vi "Brute Force Measurment SubVI.vi"(0 "Data Pin Task In":refnum<k21>, 1 "Sync Pin Task In":refnum<k21>, 2 "Write Pin Task In":refnum<k21>, 3 "Clear Pin Task In":refnum<k21>, 4 "Barcodes in":string[](array[string]), 5 "Channel # in":i32, 6 "Number of Active tubes":i32, 7 "error in (no error)":errorcluster, 9 "BoardHandle in":T1) -> (11 "Actual Voltage Level (V) 2":dbl format="%#_13g", 12 "Individual Tube Current (Nano Amps)":dbl[](array[numeric]), 13 "Failed Tubes":string[](array[string]), 14 "Data Pin Task Out":refnum<k21>, 15 "Sync Pin Task Out":refnum<k21>, 16 "Write Pin Task Out":refnum<k21>, 17 "Clear Pin Task Out":refnum<k21>, 18 "error out":errorcluster, 19 "BoardHandle out":T1)   [LabVIEW 2020]
panel:
  # "Pin in."
  # "Output pin positions"
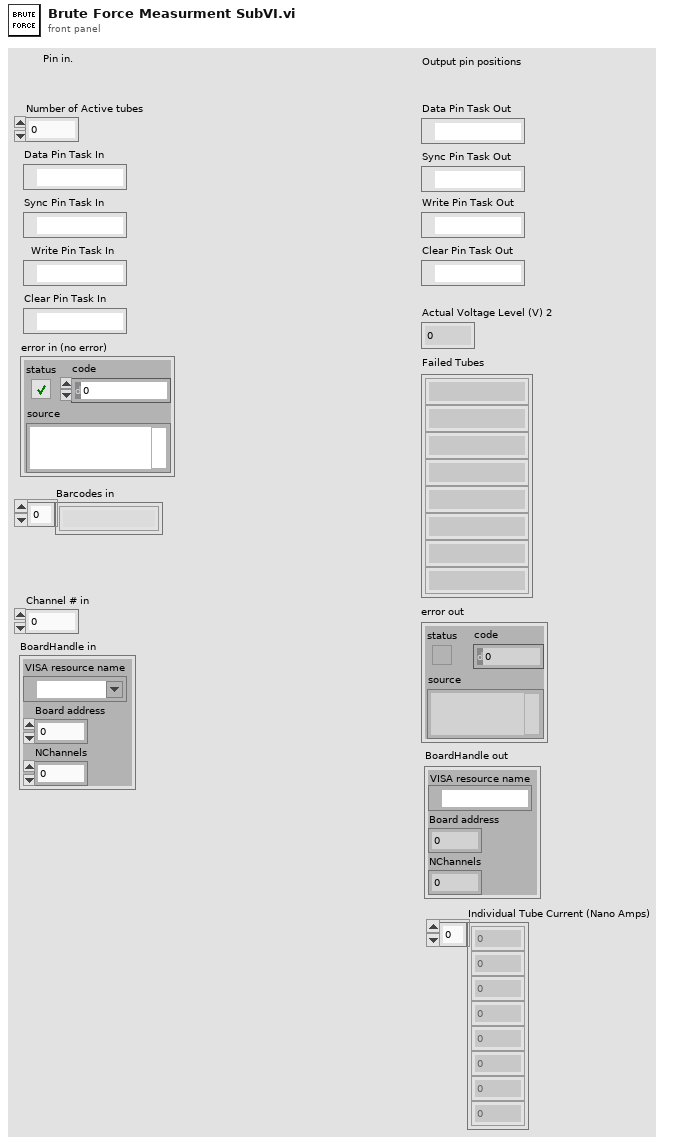
[diagram p1: front panel]
types:
  T1 = cluster{"VISA resource name":refnum<visa-resource-name>, "Board address":u8, "NChannels":u8}
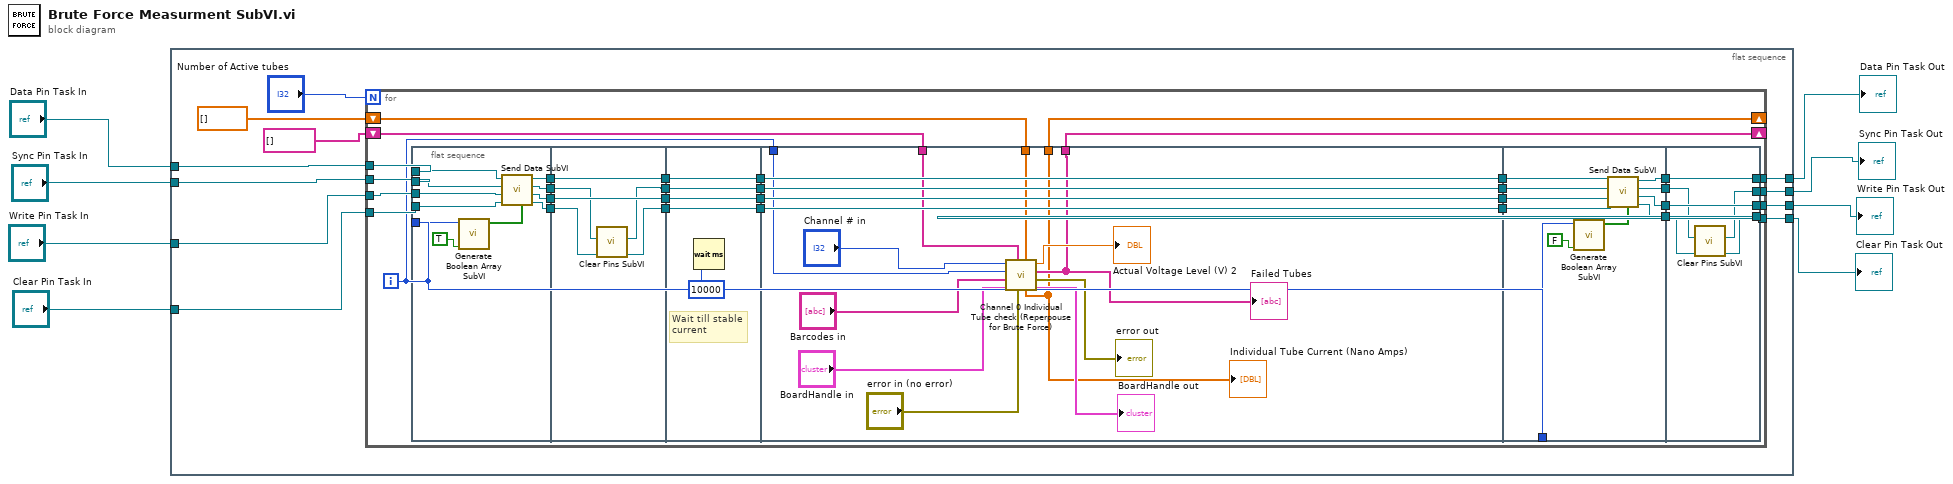
[diagram p0: block diagram]
diagram:
  n1 = flat-sequence {
    tunnel: [w18] -> w8
    tunnel: [w17] -> w7
    tunnel: [w16] -> w6
    tunnel: [w15] -> w5
    tunnel: "Data Pin Task In" -> [w14]
    tunnel: "Sync Pin Task In" -> [w13]
    tunnel: "Write Pin Task In" -> [w12]
    tunnel: "Clear Pin Task In" -> [w11]
    frame #0 {
      n2 = for {
        N: "Number of Active tubes" -> [_]
        tunnel: w14 -> [w40]
        tunnel: w13 -> [w39]
        tunnel: w12 -> [w38]
        tunnel: w11 -> [w37]
        tunnel: [w44] -> w18
        tunnel: [w43] -> w17
        tunnel: [w42] -> w16
        tunnel: [w41] -> w15
        shift-right: [w22] -> _
        shift-left: string[] [] ("Failed Tubes") -> [w23]
        shift-right: [w20] -> _
        shift-left: dbl[] [] ("Individual Tube Current In") -> [w21]
        i -> [w24]
        n3 = flat-sequence {
          tunnel: w24 -> [w63]
          tunnel: [w60] -> w52
          tunnel: [w59] -> w51
          tunnel: [w58] -> w50
          tunnel: [w57] -> w49
          tunnel: w40 -> [w56]
          tunnel: w39 -> [w55]
          tunnel: w38 -> [w54]
          tunnel: w37 -> [w53]
          tunnel: [w69] -> w36
          tunnel: w52 -> [w69]
          tunnel: [w65] -> w35
          tunnel: w51 -> [w67]
          tunnel: [w68] -> w34
          tunnel: w50 -> [w68]
          tunnel: [w64] -> w33
          tunnel: w49 -> [w66]
          tunnel: w36 -> [w74]
          tunnel: [w74] -> w32
          tunnel: w35 -> [w73]
          tunnel: [w73] -> w30
          tunnel: w34 -> [w72]
          tunnel: [w72] -> w28
          tunnel: w33 -> [w71]
          tunnel: [w71] -> w26
          tunnel: w32 -> [w90]
          tunnel: [w90] -> w31
          tunnel: w30 -> [w89]
          tunnel: [w89] -> w29
          tunnel: w28 -> [w88]
          tunnel: [w88] -> w27
          tunnel: w26 -> [w87]
          tunnel: [w87] -> w25
          tunnel: w24 -> [w79]
          tunnel: w23 -> [w78]
          tunnel: [w77] -> w22
          tunnel: w21 -> [w76]
          tunnel: [w75] -> w20
          tunnel: w24 -> [w101]
          tunnel: w31 -> [w98]
          tunnel: w29 -> [w97]
          tunnel: w27 -> [w96]
          tunnel: w25 -> [w95]
          tunnel: [w94] -> w48
          tunnel: [w93] -> w47
          tunnel: [w92] -> w46
          tunnel: [w91] -> w45
          tunnel: [w107] -> w44
          tunnel: w48 -> [w107]
          tunnel: w47 -> [w105]
          tunnel: [w106] -> w42
          tunnel: w46 -> [w106]
          tunnel: w45 -> [w104]
          tunnel: [w103] -> w43
          tunnel: [w102] -> w41
          frame #0 {
            n4 = call "Generate Boolean Array SubVI.vi"("Activate: 1\nDeactivate: 0"=TRUE, "Tube"=w63) -> ("Boolean array"=w61:bool[])  [unwired: 9 in]
            n5 = call "Send Data SubVI.vi"("Data Pin Task In"=w56, "Sync Pin Task In"=w55, "Write Pin Task In"=w54, "Clear Pin Task In"=w53, "Data"=w61) -> ("Data Pin Task Out"=w60:refnum<k21>, "Sync Pin Task Out"=w59:refnum<k21>, "Write Pin Task Out"=w58:refnum<k21>, "Clear Pin Task Out"=w57:refnum<k21>)  [unwired: 1 in]
          }
          frame #1 {
            n6 = call "Clear Pins SubVI.vi"("Clear Pin Task In"=w66, "Sync Pin Task In"=w67) -> ("Clear Pin Task Out"=w64:refnum<k21>, "Sync Pin Task Out"=w65:refnum<k21>)  [unwired: 8 in]
          }
          frame #2 {
            # "Wait till stable\ncurrent"
            n7 = Wait (ms)(milliseconds to wait=u32 10000) -> ()  [unwired: 1 out]
          }
          frame #3 {
            n8 = call "Channel 0 Individual Tube check (Reperpouse for Brute Force).vi"("Individual Tube Current In"=w76, "error in (no error)"="error in (no error)", "Failed Tubes In"=w78, "BoardHandle in"="BoardHandle in", "Barcodes in"="Barcodes in", "Tube #"=w79, "Channel # in"="Channel # in") -> ("BoardHandle out"=→"BoardHandle out":T1, "error out"=→"error out":errorcluster, "Failed Tubes"=w77:string[], "Actual Voltage Level (V) 2"=→"Actual Voltage Level (V) 2":dbl, "Individual Tube Current (Nano Amps)"=w75:dbl[])
            "Failed Tubes" <- w77
            "Individual Tube Current (Nano Amps)" <- w75
          }
          frame #4 {
            n9 = call "Generate Boolean Array SubVI.vi"("Activate: 1\nDeactivate: 0"=FALSE, "Tube"=w101) -> ("Boolean array"=w99:bool[])  [unwired: 9 in]
            n10 = call "Send Data SubVI.vi"("Data Pin Task In"=w98, "Sync Pin Task In"=w97, "Write Pin Task In"=w96, "Clear Pin Task In"=w95, "Data"=w99) -> ("Data Pin Task Out"=w94:refnum<k21>, "Sync Pin Task Out"=w93:refnum<k21>, "Write Pin Task Out"=w92:refnum<k21>, "Clear Pin Task Out"=w91:refnum<k21>)  [unwired: 1 in]
          }
          frame #5 {
            n11 = call "Clear Pins SubVI.vi"("Clear Pin Task In"=w104, "Sync Pin Task In"=w105) -> ("Clear Pin Task Out"=w102:refnum<k21>, "Sync Pin Task Out"=w103:refnum<k21>)  [unwired: 8 in]
          }
        }
      }
    }
  }
  "Clear Pin Task Out" <- w5
  "Data Pin Task Out" <- w8
  "Write Pin Task Out" <- w6
  "Sync Pin Task Out" <- w7
